vi "List Compatible Ctls.vi"(11 "UIP In":refnum<class "TipStripUIP.lvclass">) -> (2 "Compatible Ctls":string[](array[string]), 3 "UIP Out":refnum<class "TipStripUIP.lvclass">)   [LabVIEW 2020, in "UIM.lvlib" / "TipStripUIP.lvclass"]
doc: "Overwrite this method in your child UIPs to provide a custom list of vi server control classes compatible with that UIP."
uses:
  TipStripUIP.lvclass
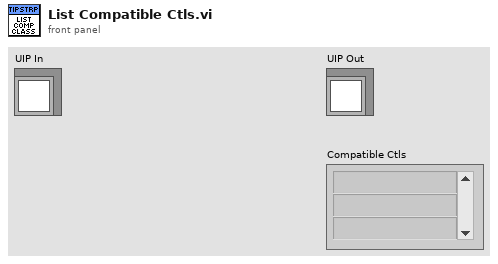
[diagram p1: front panel]
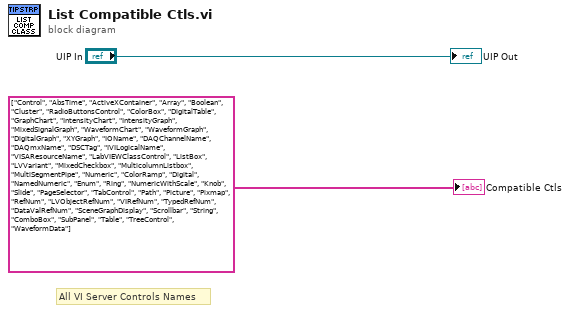
[diagram p0: block diagram]
diagram:
  # "All VI Server Controls Names"
  "Compatible Ctls" <- string[] ["Control", "AbsTime", "ActiveXContainer", "Array", "Boolean", "Cluster", "RadioButtonsControl", "ColorBox", "DigitalTable", "GraphChart", "IntensityChart", "IntensityGraph", "MixedSignalGraph", "WaveformChart", "WaveformGraph", "DigitalGraph", "XYGraph", "IOName", "DAQChannelName", "DAQmxName", "DSCTag", "IVILogicalName", "VISAResourceName", "LabVIEWClassControl", "ListBox", "LVVariant", "MixedCheckbox", "MulticolumnListbox", "MultiSegmentPipe", "Numeric", "ColorRamp", "Digital", "NamedNumeric", "Enum", "Ring", "NumericWithScale", "Knob", "Slide", "PageSelector", "TabControl", "Path", "Picture", "Pixmap", "RefNum", "LVObjectRefNum", "VIRefNum", "TypedRefNum", "DataValRefNum", "SceneGraphDisplay", "Scrollbar", "String", "ComboBox", "SubPanel", "Table", "TreeControl", "WaveformData"]
  "UIP Out" <- "UIP In"
